vi "Launcher.vi"() -> ()   [LabVIEW 2019, in "Package Builder.lvlib"]
uses:
  Package Builder.lvlib
  TypeDefs/Application Launcher States.ctl
  TypeDefs/Application Launcher IDC.ctl
  <vilib>/Utility/sysdir.llb/System Directory Type.ctl
  <vilib>/National Instruments/NIPM API (Beta)/NIPM_API.lvlib
panel:
  out "error IO":errorcluster
  out "Progress":u8(slide) scale=0.0..5.0
  out "Action":string caption="String"
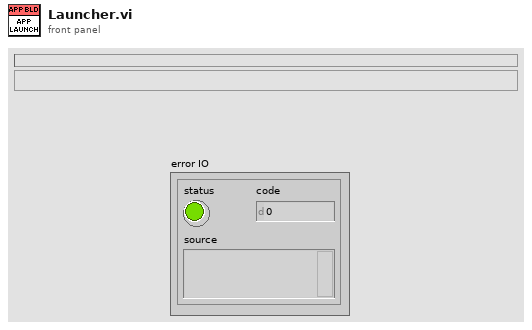
[diagram p1: front panel]
types:
  T1 = typedef "Package Builder.lvlib/Application Launcher States.ctl" = enum16{"Launch Application", "Install Packages", "Update Packages", "Check Installed Packages", "Register Feed", "Check Feed", "Shutdown", "Initialize", "Error"}
  T2 = enum32{"Invalid", "Standard", "Closed", "Hidden", "Minimized", "Maximized"}
  T3 = typedef "Package Builder.lvlib/Application Launcher IDC.ctl" = cluster{"Feed URL":string, "Feed Name":string, "Package Name":string, "Target Application Path":path}
  T4 = typedef "NIPM_API.lvlib/feed.ctl" = cluster{"Name":string, "URI":string}
  T5 = enum16{"Always On", "Always Off", "Off While Running"}
  T6 = typedef "System Directory Type.ctl" = i32
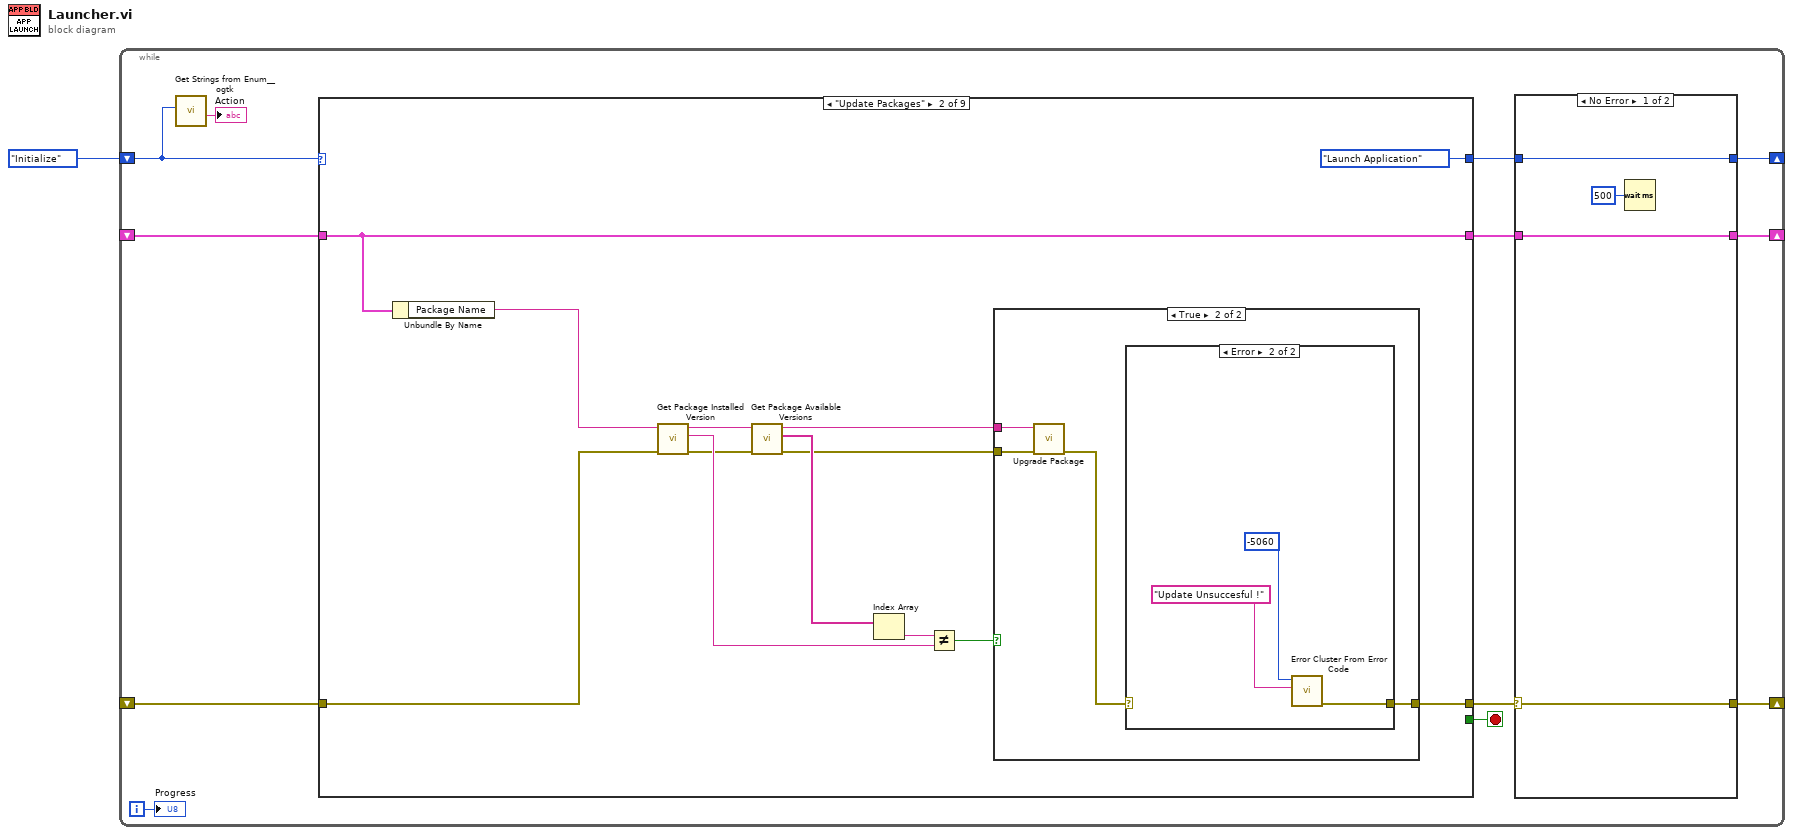
[diagram p0: block diagram]
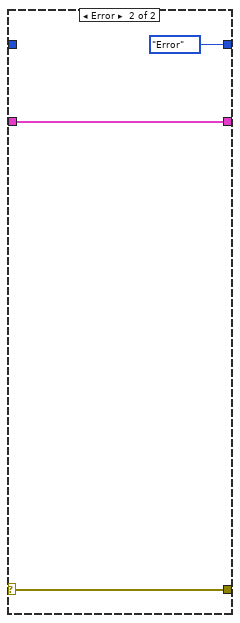
[diagram p2: hidden frame]
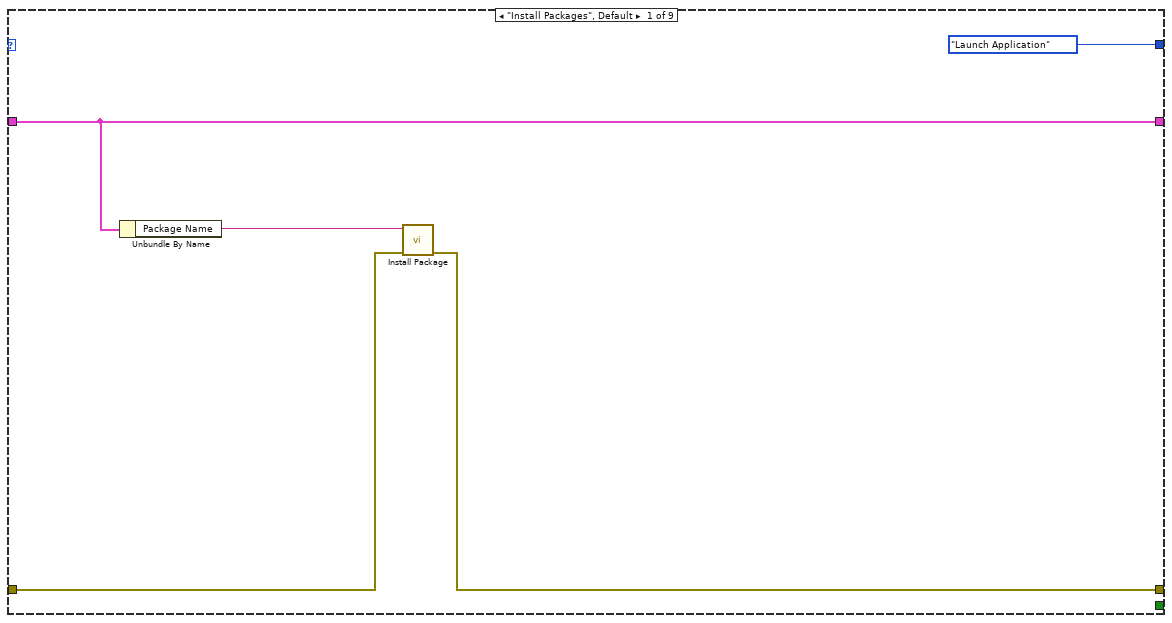
[diagram p3: hidden frame]
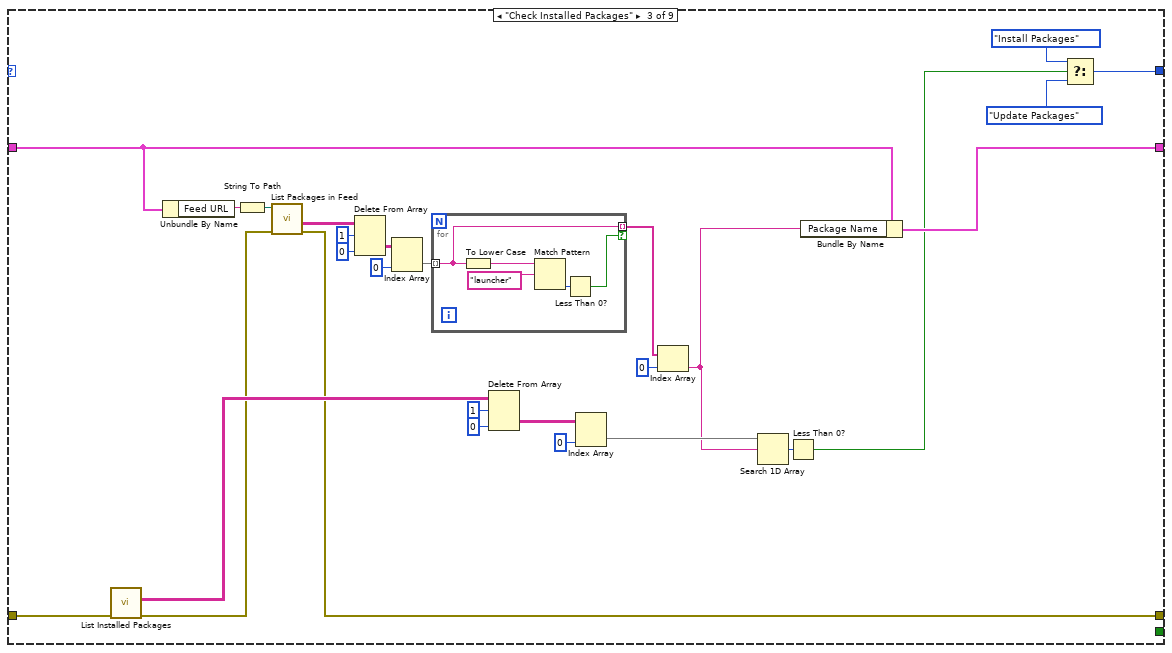
[diagram p6: hidden frame]
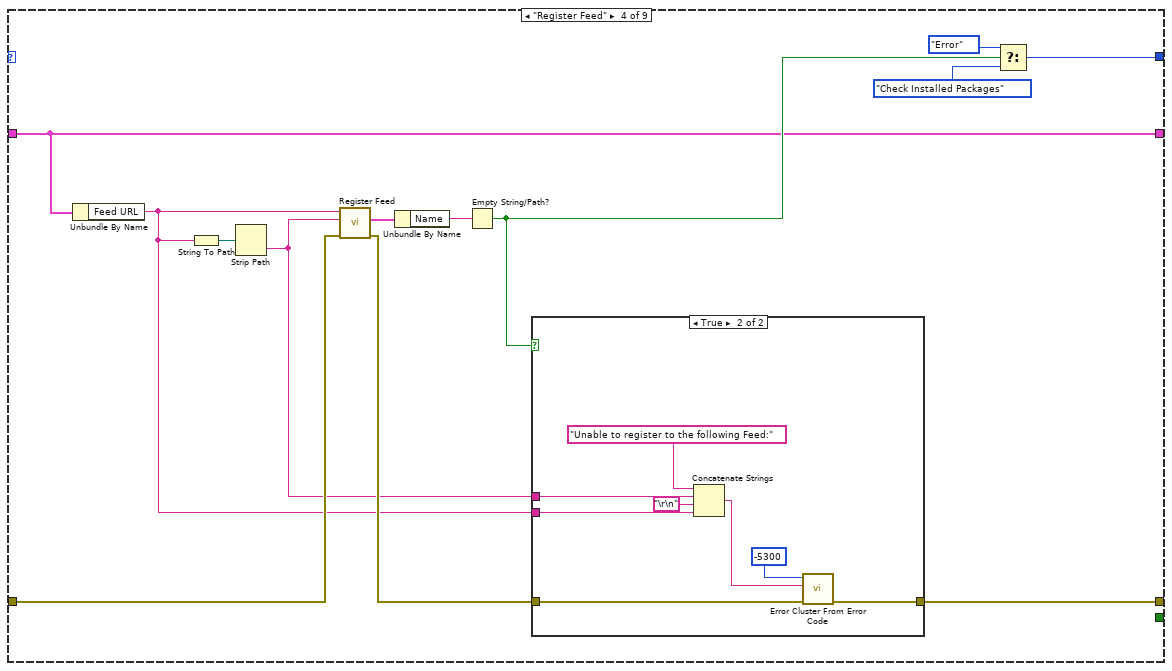
[diagram p7: hidden frame]
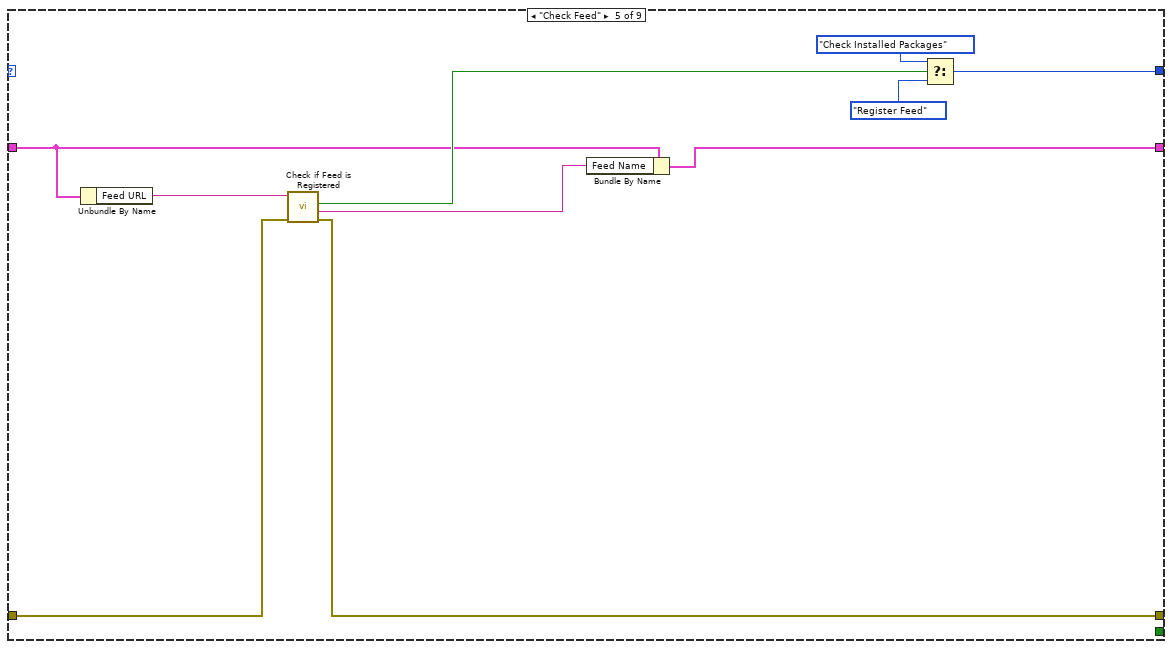
[diagram p9: hidden frame]
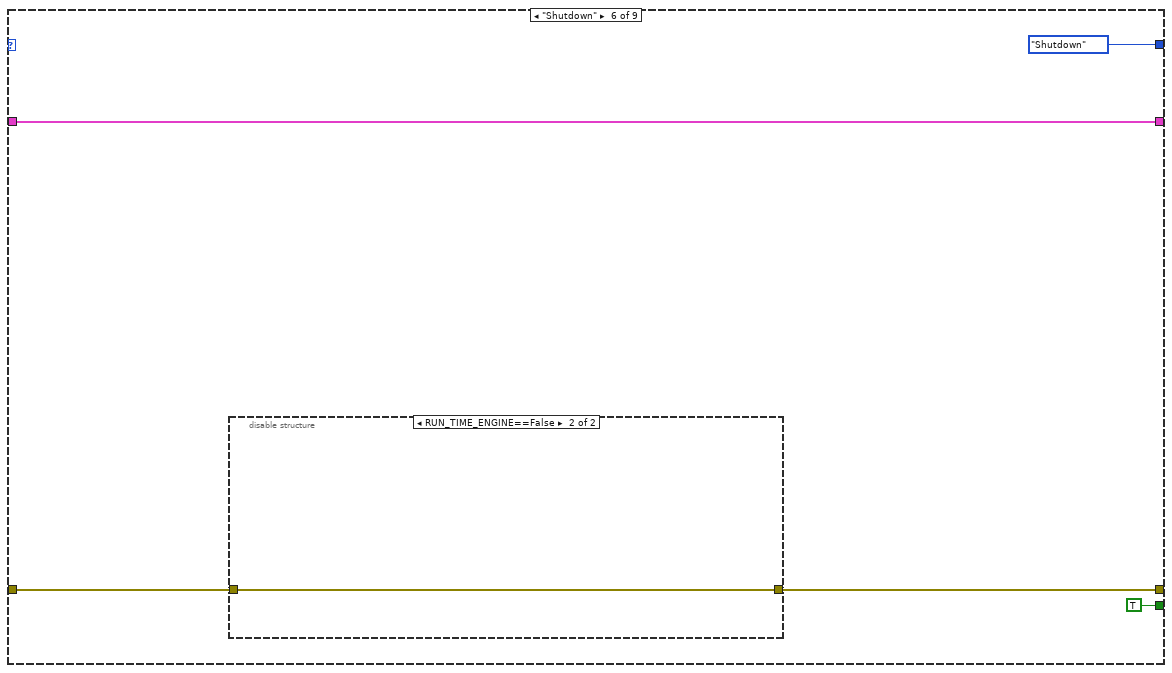
[diagram p10: hidden frame]
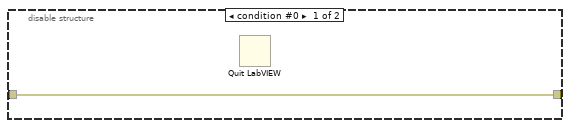
[diagram p11: hidden frame]
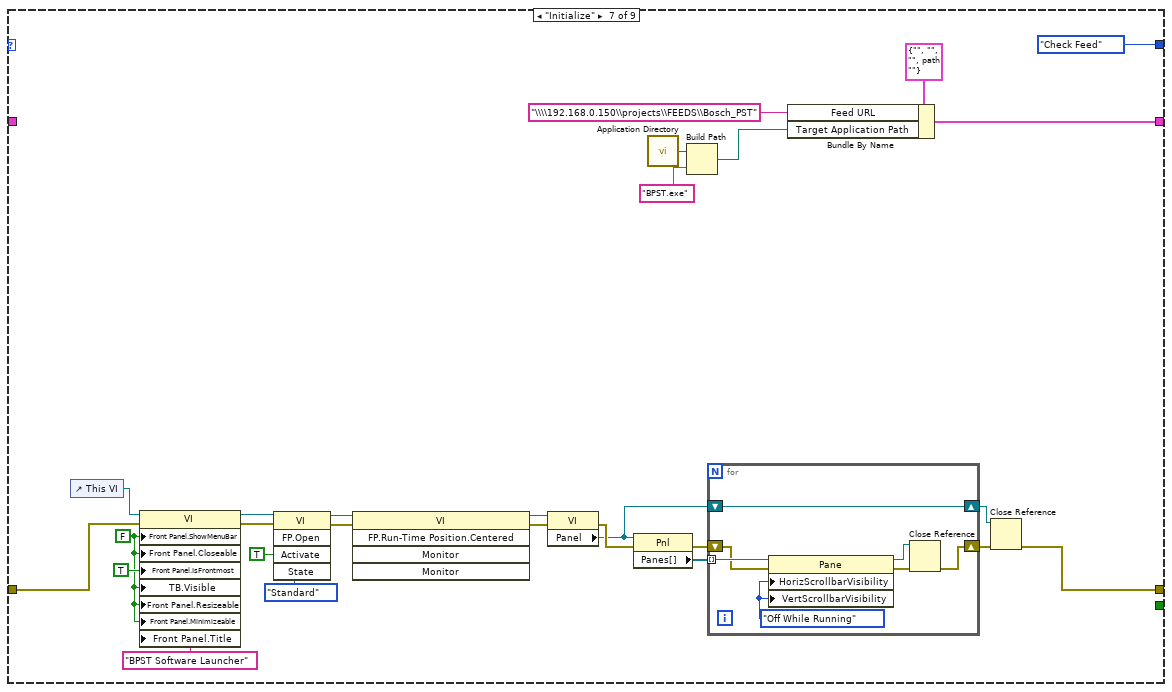
[diagram p12: hidden frame]
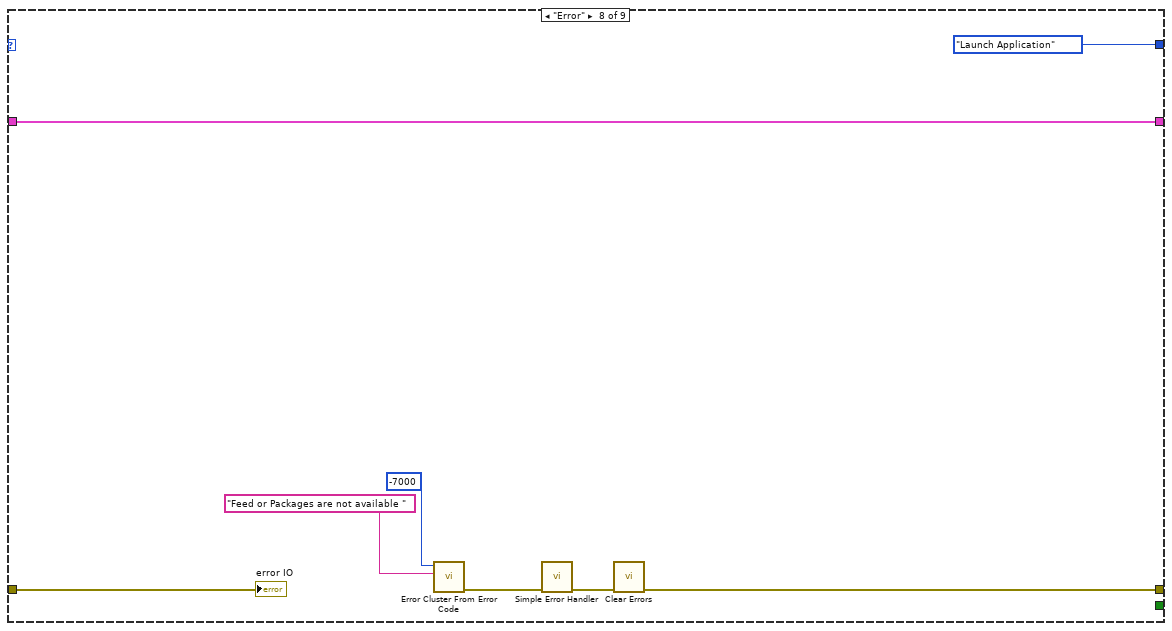
[diagram p13: hidden frame]
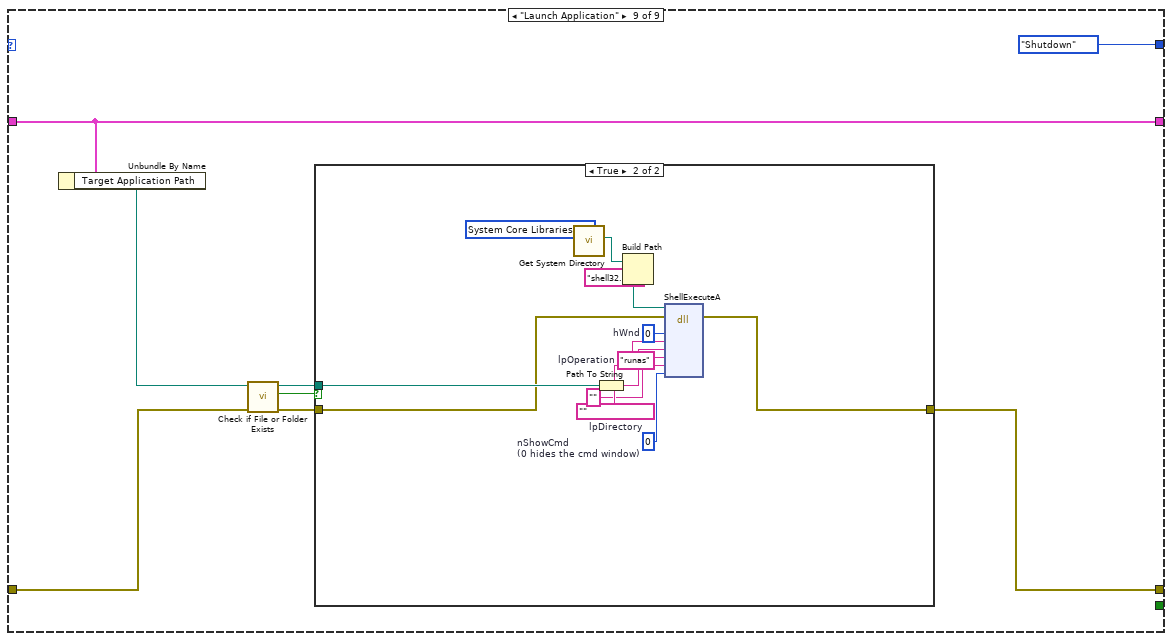
[diagram p14: hidden frame]
diagram:
  n1 = while {
    shift-right: [w12] -> _
    shift-left: _ -> [w11]
    shift-right: [w6] -> _
    shift-left: _ -> [w5]
    shift-right: [w8] -> _
    shift-left: Application_Launcher_States."Initialize" -> [w4]
    i -> [w2]
    stop <- w10 stop-if-true
    n2 = call <userlib>:"Get Strings from Enum__ogtk.vi"("Enum"=w4) -> ("String Value"=→"Action":string)  [unwired: 7 in, 3 out]
    n3 = case shown="\"Update Packages\"" w4 {
      tunnel: [w23 w33 w50 w85 w104 w112 w123 w157 w166] -> w13
      tunnel: w11 -> [w24 w38 w71 w92 w110 w113 w133 w153 w163]
      tunnel: [_ _ _ _ _ TRUE _ _ _] -> w10
      tunnel: [Application_Launcher_States."Launch Application" Application_Launcher_States."Launch Application" w74 w89 w108 Application_Launcher_States."Shutdown" Application_Launcher_States."Check Feed" Application_Launcher_States."Launch Application" Application_Launcher_States."Shutdown"] -> w9
      tunnel: [w22 w32 w53 w83 w105 w114 w142 w159 w167] -> w7
      tunnel: w5 -> [w22 w32 w55 w83 w107 w114 _ w159 w167]
      frame "Install Packages", Default {
        n4 = Unbundle By Name(w22) -> ("Package Name"=w25:string)
        n5 = call <vilib>:"Install Package.vi"("error in"=w24, "package name"=w25) -> ("error out"=w23:errorcluster)  [unwired: 7 in, 2 out]
      }
      frame "Update Packages" {
        n6 = Unbundle By Name(w32) -> ("Package Name"=w37:string)
        n7 = call <vilib>:"Get Package Installed Version.vi"("error in"=w38, "package name"=w37) -> ("error out"=w26:errorcluster, "installed version"=w30:string, "package name out"=w27:string)  [unwired: 6 in, 1 out]
        n8 = call <vilib>:"Get Package Available Versions.vi"("error in"=w26, "package name"=w27) -> ("error out"=w29:errorcluster, "versions"=w36:string[], "package name out"=w28:string)  [unwired: 7 in]
        n9 = Index Array(array=w36) -> (element=w35:string)  [unwired: 1 in]
        n10 = Not Equal?(x=w35, y=w30) -> (x != y?=w34:bool)
        n11 = case shown="True" w34 {
          tunnel: w29 -> [w39 w43]
          tunnel: w28 -> [_ w42]
          tunnel: [w39 w40] -> w33
          frame False {
          }
          frame True {
            n12 = call <vilib>:"Upgrade Package.vi"("error in"=w43, "package name"=w42) -> ("error out"=w41:errorcluster)  [unwired: 6 in, 3 out]
            n13 = case shown="Error" w41 {
              selector: w41 -> [w44 _]
              tunnel: [w44 w47] -> w40
              frame No Error {
              }
              frame Error {
                n14 = call <vilib>:"Error Cluster From Error Code.vi"("error message (\"\")"="Update Unsuccesful !" ("error message (\"\")"), "error code (0)"=-5060) -> ("error out"=w47:errorcluster)  [unwired: 7 in]
              }
            }
          }
        }
      }
      frame "Check Installed Packages" {
        n15 = call <vilib>:"List Installed Packages.vi"("error in"=w71) -> ("error out"=w51:errorcluster, "installed packages"=w70:string[][])  [unwired: 9 in]
        n16 = Unbundle By Name(w55) -> ("Feed URL"=w67:string)
        n17 = String To Path(string=w67) -> (path=w66:path)
        n18 = call <vilib>:"List Packages in Feed.vi"("error in"=w51, "feed folderpath in"=w66) -> ("error out"=w50:errorcluster, "package names and versions"=w65:string[][])  [unwired: 6 in, 2 out]
        n19 = Delete From Array(array=w65, length=1, index (col)=0 ("disabled index (col)")) -> (deleted portion=w62:string[][])  [unwired: 1 in, 1 out]
        n20 = Index Array(array=w62, index (col)=0 ("disabled index (col)")) -> (element=w60:string[])  [unwired: 1 in]
        n21 = for {
          tunnel: w60 -> [w77] mode=indexing
          tunnel: [w77] -> w57 mode=indexing if=w75
          n22 = To Lower Case(string=w77) -> (all lower case string=w78:string)
          n23 = Match Pattern(string=w78, regular expression="launcher") -> (offset past match=w76:i32)  [unwired: 1 in, 3 out]
          n24 = Less Than 0?(x=w76) -> (x < 0?=w75:bool)
        }
        n25 = Delete From Array(array=w70, length=1, index (col)=0 ("disabled index (col)")) -> (deleted portion=w61:string[][])  [unwired: 1 in, 1 out]
        n26 = Index Array(array=w61, index (col)=0 ("disabled index (col)")) -> (element=w59:string[])  [unwired: 1 in]
        n27 = Index Array(array=w57, index=0) -> (element=w54:string)
        n28 = Search 1D Array(1D array=w59, element=w54) -> (index of element=w58:i32)  [unwired: 1 in]
        n29 = Less Than 0?(x=w58) -> (x < 0?=w52:bool)
        n30 = Bundle By Name(cluster=w55, "Package Name"=w54) -> (w53:T3)
        n31 = Select(t=Application_Launcher_States."Install Packages", s=w52, f=Application_Launcher_States."Update Packages") -> (s? t:f=w74:T1)
      }
      frame "Register Feed" {
        n32 = Unbundle By Name(w83) -> ("Feed URL"=w81:string)
        n33 = String To Path(string=w81) -> (path=w82:path)
        n34 = Strip Path(path=w82) -> (name=w80:string)  [unwired: 1 out]
        n35 = call <vilib>:"Register Feed.vi"("error in"=w92, "feed name"=w80, "feed URI"=w81) -> ("error out"=w86:errorcluster, "registered feed"=w91:T4)  [unwired: 7 in]
        n36 = Unbundle By Name(w91) -> ("Name"=w90:string)
        n37 = Empty String/Path?(string/path=w90) -> (empty?=w84:bool)
        n38 = case shown="True" w84 {
          tunnel: w86 -> [w93 w101]
          tunnel: [w93 w100] -> w85
          tunnel: w81 -> [_ w96]
          tunnel: w80 -> [_ w94]
          frame False {
          }
          frame True {
            n39 = Concatenate Strings("Unable to register to the following Feed:" ("string"), w94, "\r\n", w96) -> (w95:string)
            n40 = call <vilib>:"Error Cluster From Error Code.vi"("error in (no error)"=w101, "error message (\"\")"=w95, "error code (0)"=-5300) -> ("error out"=w100:errorcluster)  [unwired: 6 in]
          }
        }
        n41 = Select(t=Application_Launcher_States."Error", s=w84, f=Application_Launcher_States."Check Installed Packages") -> (s? t:f=w89:T1)
      }
      frame "Check Feed" {
        n42 = Unbundle By Name(w107) -> ("Feed URL"=w111:string)
        n43 = call <vilib>:"Check if Feed is Registered.vi"("error in"=w110, "feed URI"=w111) -> ("error out"=w104:errorcluster, "feed name"=w106:string, "feed URI registered?"=w109:bool)  [unwired: 6 in, 1 out]
        n44 = Bundle By Name(cluster=w107, "Feed Name"=w106) -> (w105:T3)
        n45 = Select(t=Application_Launcher_States."Check Installed Packages", s=w109, f=Application_Launcher_States."Register Feed") -> (s? t:f=w108:T1)
      }
      frame "Shutdown" {
        n46 = disable-structure shown="RUN_TIME_ENGINE==False" {
          disable-tunnel: w113 -> [w117 w118]
          disable-tunnel: [w117 w118] -> w112
          frame condition #0 {
            n47 = Quit LabVIEW() -> ()  [unwired: 1 in]
          }
          frame condition #1 (active) {
          }
        }
      }
      frame "Initialize" {
        w122 = FALSE ("Front Panel Window:Show Menu Bar")
        n48 = control-ref of="This VI"() -> (w138:refnum<vi>)
        n49 = property class="VI"(reference=w138, error in=w133, "Front Panel.ShowMenuBar"=w122, "Front Panel.Closeable"=w122, "Front Panel.IsFrontmost"=TRUE ("Front Panel Window:Is Frontmost"), "TB.Visible"=w122, "Front Panel.Resizeable"=w122, "Front Panel.Minimizeable"=w122, "Front Panel.Title"="BPST Software Launcher" ("Front Panel Window:Title")) -> (reference out=w137:refnum<vi>, error out=w136:errorcluster)
        n50 = invoke class="VI" method="FP.Open"(reference=w137, error in=w136, "Activate"=TRUE ("Activate?"), "State"=T2."Standard") -> (reference out=w139:refnum<vi>, error out=w140:errorcluster)  [unwired: 1 in, 3 out]
        n51 = invoke class="VI" method="FP.Run-Time Position.Centered"(reference=w139, error in=w140) -> (reference out=w131:refnum<vi>, error out=w129:errorcluster)  [unwired: 3 in, 3 out]
        n52 = property class="VI"(reference=w131, error in=w129) -> (error out=w128:errorcluster, "Panel"=w125:refnum<vi>)  [unwired: 1 out]
        n53 = property class="Pnl"(reference=w125, error in=w128) -> (error out=w127:errorcluster, "Panes[]"=w130:refnum<vi>[])  [unwired: 1 out]
        n54 = call <vilib>:"Application Directory.vi"() -> ("Application Directory"=w120:path)
        n55 = Build Path(base path=w120, name or relative path="BPST.exe") -> (appended path=w132:path)
        n56 = for {
          tunnel: w130 -> [w152] mode=indexing
          shift-right: [w147] -> w126
          shift-left: w127 -> [w150]
          shift-right: [w146] -> w124
          shift-left: w125 -> [w146]
          w151 = T5."Off While Running" ("Horizontal Scrollbar Visibility")
          n57 = property class="Pane"(reference=w152, error in=w150, "HorizScrollbarVisibility"=w151, "VertScrollbarVisibility"=w151) -> (reference out=w148:refnum<vi>, error out=w149:errorcluster)
          n58 = Close Reference(reference=w148, error in (no error)=w149) -> (error out=w147:errorcluster)
        }
        n59 = Bundle By Name(cluster=T3 {"Feed URL"="", "Feed Name"="", "Package Name"="", "Target Application Path"=path ""} ("Internal Data Cluster"), "Feed URL"="\\\\192.168.0.150\\projects\\FEEDS\\Bosch_PST" ("feed URI"), "Target Application Path"=w132) -> (w142:T3)
        n60 = Close Reference(reference=w124, error in (no error)=w126) -> (error out=w123:errorcluster)
      }
      frame "Error" {
        n61 = call <vilib>:"Error Cluster From Error Code.vi"("error message (\"\")"="Feed or Packages are not available " ("error message (\"\")"), "error code (0)"=-7000) -> ("error out"=w156:errorcluster)  [unwired: 7 in]
        n62 = call <vilib>:"Simple Error Handler.vi"("error in (no error)"=w156) -> ("error out"=w158:errorcluster)  [unwired: 4 in, 4 out]
        n63 = call <vilib>:"Clear Errors.vi"("error in (no error)"=w158) -> ("error out"=w157:errorcluster)  [unwired: 5 in, 1 out]
        "error IO" <- w153
      }
      frame "Launch Application" {
        n64 = Unbundle By Name(w167) -> ("Target Application Path"=w165:path)
        n65 = call <vilib>:"Check if File or Folder Exists.vi"("error in (no error)"=w163, "path"=w165) -> ("error out"=w162:errorcluster, "file or folder exists?"=w161:bool, "dup path"=w164:path)  [unwired: 7 in]
        n66 = case shown="True" w161 {
          tunnel: [w169 w172] -> w166
          tunnel: w164 -> [_ w171]
          tunnel: w162 -> [w169 w170]
          frame False {
          }
          frame True {
            w174 = 0  # nShowCmd (0 hides the cmd window)
            w175 = ""  # lpDirectory
            w177 = "runas"  # lpOperation
            w178 = 0  # hWnd
            w182 = T6 9 items=["User Home"=0, "User Desktop"=1, "User Documents"=2, "User Application Data"=3, "User Preferences"=4, "User Temporary"=5, "Public Documents"=6, "Public Application Data"=7, "Public Preferences"=8, "Public Cache"=13, "System Core Libraries"=9, "System Installed Libraries"=10, "Application Files"=11, "Boot Volume Root"=12] ("system directory type")
            n67 = call <vilib>:"Get System Directory.vi"("system directory type"=w182) -> ("system directory"=w181:path)  [unwired: 10 in]
            n68 = Path To String(path=w171) -> (string=w176:string)
            n69 = Build Path(base path=w181, name or relative path="shell32.dll") -> (appended path=w179:path)
            n70 = dll-call lib="C:/Windows/System32/shell32.dll" fn="ShellExecuteA"(path in=w179, error in=w170, "hWnd"=w178, "lpOperation"=w177, "lpFile"=w176, "lpParameters"="", "lpDirectory"=w175, "nShowCmd"=w174) -> (error out=w172:errorcluster)  [unwired: 8 in, 1 out]
          }
        }
      }
    }
    n71 = case shown="No Error" w13 {
      selector: w13 -> [w17 w19]
      tunnel: [w17 w19] -> w12
      tunnel: w9 -> [w16 _]
      tunnel: [w16 Application_Launcher_States."Error"] -> w8
      tunnel: [w15 w18] -> w6
      tunnel: w7 -> [w15 w18]
      frame No Error {
        n72 = Wait (ms)(milliseconds to wait=u32 500) -> ()  [unwired: 1 out]
      }
      frame Error {
      }
    }
    "Progress" <- w2
  }
